vi "NIVS Sys Def Root Read.vi"(4 "error in (no error)":errorcluster, 6 "Container State":T4, 7 "Display State In":T1={"Initialization"=TRUE, "Show In and out values"=TRUE, "Show Highliting"=TRUE, "Open Plot"=FALSE, "Format String"="%10_4g", "Limits"={"Min X"=-inf, "Max X"=inf, "MaxDiff X"=inf, "MaxGrad X"=inf, "Min Y"=-inf, "Max Y"=inf, "MaxDiff Y"=inf}, "Vertical Scrollbar"=FALSE, "Data"={"X"=[0.0, 5.0], "Y"=[0.0, 100.0]}, "Undo Avaliable"=FALSE, "NIVS.System Definition Root"=refnum, "Selected Parameter"="", "Selected Working Pt"=[], "X"=0.0, "Y"=0.0, "Row Axis"=""}) -> (0 "error out":errorcluster, 2 "Value":refnum<k24>, 3 "Display State Out":T1={"Initialization"=TRUE, "Show In and out values"=TRUE, "Show Highliting"=TRUE, "Open Plot"=FALSE, "Format String"="%10_4g", "Limits"={"Min X"=-inf, "Max X"=inf, "MaxDiff X"=inf, "MaxGrad X"=inf, "Min Y"=-inf, "Max Y"=inf, "MaxDiff Y"=inf}, "Vertical Scrollbar"=FALSE, "Data"={"X"=[0.0, 5.0], "Y"=[0.0, 100.0]}, "Undo Avaliable"=FALSE, "NIVS.System Definition Root"=refnum, "Selected Parameter"="", "Selected Working Pt"=[], "X"=0.0, "Y"=0.0, "Row Axis"=""})   [LabVIEW 2011, in "TBL1D.xctl"]
uses:
  TBL1D.xctl
  <vilib>/_xctls/Container State.ctl
  State TBL1D.ctl
  Limits TBL1D.ctl
  Data TBL1D.ctl
  NationalInstruments.VeriStand.SystemStorage
  <vilib>/_xctls/XControlSupport.lvlib
panel:
  # "Replace the Value Indicator below with an Indicator of desired type.\nDo not remove this Indicator or the others from the connector pane. \nDo not change the connector pane pattern.\nThe Value Indicator should always be the second terminal from top on the output side in the connector pane."
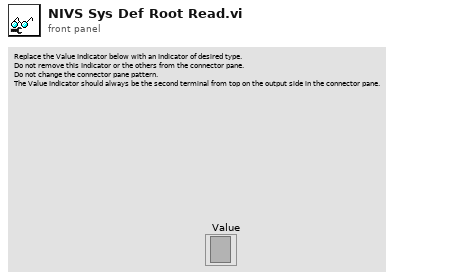
[diagram p1: front panel]
types:
  T1 = typedef "TBL1D.xctl/State TBL1D.ctl" = cluster{"Initialization":bool, "Show In and out values":bool, "Show Highliting":bool, "Open Plot":bool, "Format String":string, "Limits":T2, "Vertical Scrollbar":bool, "Data":T3, "Undo Avaliable":bool, "NIVS.System Definition Root":refnum<k24>, "Selected Parameter":string, "Selected Working Pt":string[], "X":sgl, "Y":sgl, "Row Axis":string}
  T2 = typedef "TBL1D.xctl/Limits TBL1D.ctl" = cluster{"Min X":sgl, "Max X":sgl, "MaxDiff X":sgl, "MaxGrad X":sgl, "Min Y":sgl, "Max Y":sgl, "MaxDiff Y":sgl}
  T3 = typedef "TBL1D.xctl/Data TBL1D.ctl" = cluster{"X":sgl[], "Y":sgl[]}
  T4 = typedef "XControlSupport.lvlib/Container State.ctl" = cluster{"Indicator?":bool, "Run Mode?":bool, " Refnum":refnum<vi>}
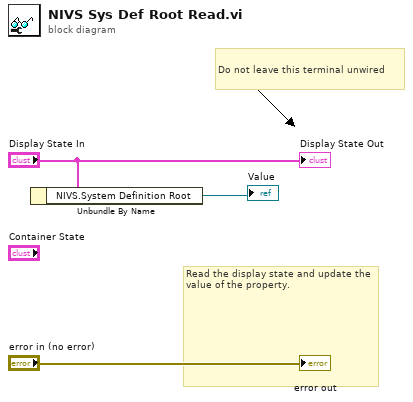
[diagram p0: block diagram]
diagram:
  # "Do not leave this terminal unwired"
  # "Read the display state and update the value of the property."
  n1 = Unbundle By Name("Display State In") -> ("NIVS.System Definition Root"=→"Value":refnum<k24>)
  "error out" <- "error in (no error)"
  "Display State Out" <- "Display State In"
